vi "FSF.vi"(0 "System no.":i32=1 min=1 max=4 step=1, 1 "Affected axis":string, 2 "Force value 1":dbl format="%.6f", 3 "Position offset":dbl format="%.6f", 4 "No.of digits":i16=4, 5 "error in":errorcluster, 7 "Use Force value 2?":bool, 9 "Force value 2":dbl format="%.6f") -> (19 "error out":errorcluster)   [LabVIEW 2020]
doc: "Performs a find surface procedure.\nApproaches the surface with force value 1. After making contact with the surface the parameter for surface position is set. The parameter for pre-position is set accordingly to the value of position offset.\n\nC-413:"
panel:
  # "Starts find surface procedure for selected axis"
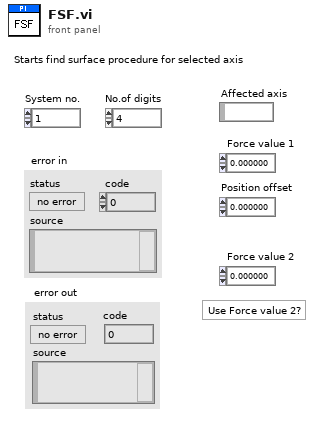
[diagram p1: front panel]
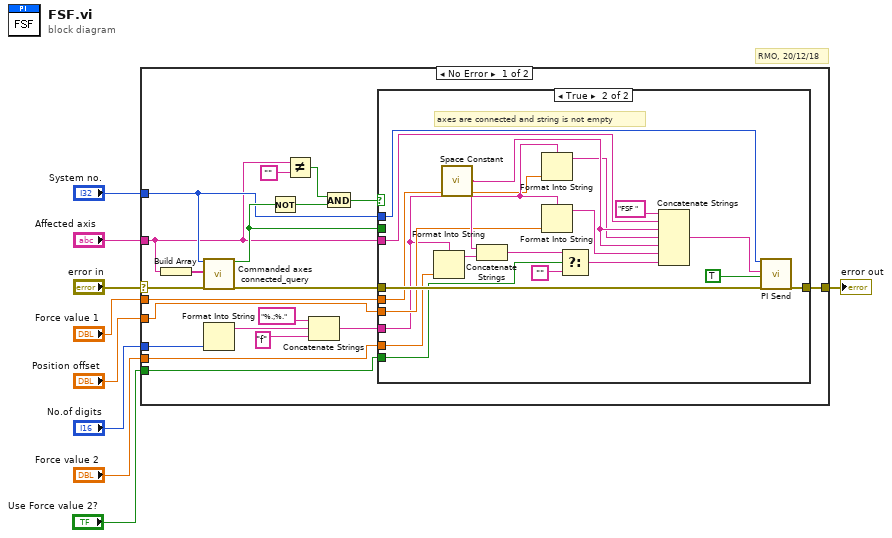
[diagram p0: block diagram]
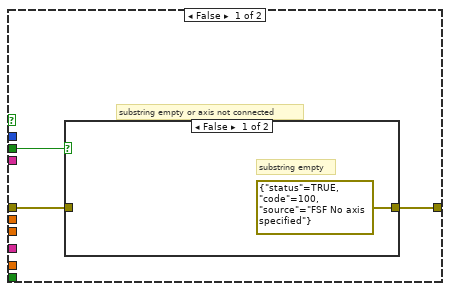
[diagram p2: hidden frame]
diagram:
  # "RMO, 20/12/18"
  n1 = case shown="No Error" "error in" {
    selector: "error in" -> [w10 w54]
    tunnel: [w29 w54] -> w9
    tunnel: "System no." -> [w19 _]
    tunnel: "Affected axis" -> [w18 _]
    tunnel: "Force value 1" -> [w22 _]
    tunnel: "Position offset" -> [w21 _]
    tunnel: "Force value 2" -> [w20 _]
    tunnel: "No.of digits" -> [w11 _]
    tunnel: "Use Force value 2?" -> [w16 _]
    frame No Error {
      n2 = Build Array(w18) -> (w17:string[])
      n3 = call "Commanded axes connected_query.vi"("System no."=w19, "Commanded axes"=w17, "error in"=w10) -> ("Controller error"=w25:bool, "error out"=w27:errorcluster)  [unwired: 1 in, 14 out]
      n4 = Format Into String(w11) -> (resulting string=w15:string)  [unwired: 3 in, 1 out]
      n5 = Not(x=w25) -> (.not. x?=w24:bool)
      n6 = Not Equal?(x=w18, y="") -> (x != y?=w26:bool)
      n7 = Concatenate Strings("%.;%." ("Format String"), w15, "f" ("Format String")) -> (w12:string)
      n8 = And(x=w26, y=w24) -> (x .and. y?=w23:bool)
      n9 = case shown="True" w23 {
        tunnel: [w32 w50] -> w29
        tunnel: w27 -> [w30 w51]
        tunnel: w25 -> [w31 _]
        tunnel: w19 -> [_ w49]
        tunnel: w18 -> [_ w48]
        tunnel: w22 -> [_ w37]
        tunnel: w21 -> [_ w42]
        tunnel: w20 -> [_ w38]
        tunnel: w12 -> [_ w39]
        tunnel: w16 -> [_ w36]
        frame False {
          # "substring empty or axis not connected"
          n10 = case shown="False" w31 {
            tunnel: [errorcluster {"status"=TRUE, "code"=100, "source"="FSF No axis specified"} ("error out") w34] -> w32
            tunnel: w30 -> [_ w34]
            frame False {
              # "substring empty"
            }
            frame True {
              # "commanded axis not connected"
            }
          }
        }
        frame True {
          # "axes are connected and string is not empty"
          n11 = Format Into String(format string=w39, w38) -> (resulting string=w40:string)  [unwired: 2 in, 1 out]
          n12 = call "Space Constant.vi"() -> ("String"=w44:string)
          n13 = Concatenate Strings(w44, w40) -> (w47:string)
          n14 = Format Into String(format string=w39, w37) -> (resulting string=w43:string)  [unwired: 2 in, 1 out]
          n15 = Format Into String(format string=w39, w42) -> (resulting string=w41:string)  [unwired: 2 in, 1 out]
          n16 = Select(t=w47, s=w36, f="" ("Empty String Constant")) -> (s? t:f=w45:string)
          n17 = Concatenate Strings("FSF ", w48, w44, w43, w44, w41, w45) -> (w35:string)
          n18 = call "PI Send.vi"("System no."=w49, "String to send"=w35, "Attach termination char.?"=TRUE ("Attach Linefeed?"), "error in"=w51) -> ("error out"=w50:errorcluster)  [unwired: 2 in, 13 out]
        }
      }
    }
    frame Error {
    }
  }
  "error out" <- w9
